vi "Config2Double.vi"(10 "Numeric in":u32, 11 "Config Address":T1 items=["ID", "Mode", "Baudrate", "Homing Offset", "Id P gain", "Id I gain", "Id D gain", "Iq P gain", "Iq I gain", "Iq D gain", "Velo P gain", "Velo I gain", "Velo D gain", "Posi P gain", "Posi I gain", "Posi D gain", "DirectForce P", "DirectForce I", "DirectForce D", "Limit Id Max", "Limit Iq Max", "Limit Velo Max", "Limit Posi Min", "Limit Posi Max", "Voltage Min", "Voltage Max", "Watchdog", "Temperature Low", "Temperature High"]) -> (3 "Numeric out":dbl)   [LabVIEW 2016, in "REV_2.lvlib"]
uses:
  REV_2.lvlib
  REV2_Config_Addr.ctl
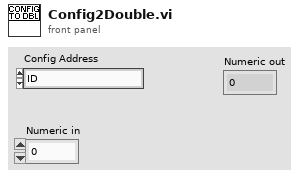
[diagram p1: front panel]
types:
  T1 = typedef "REV_2.lvlib/REV2_Config_Addr.ctl" = u8
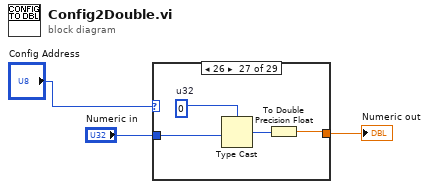
[diagram p0: block diagram]
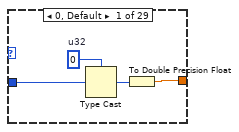
[diagram p2: hidden frame]
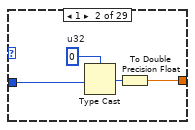
[diagram p3: hidden frame]
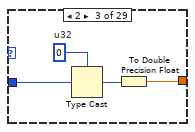
[diagram p4: hidden frame]
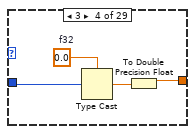
[diagram p5: hidden frame]
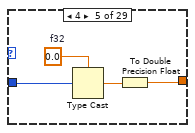
[diagram p6: hidden frame]
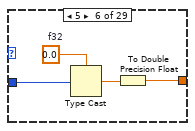
[diagram p7: hidden frame]
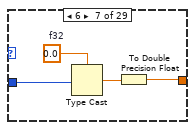
[diagram p8: hidden frame]
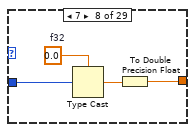
[diagram p9: hidden frame]
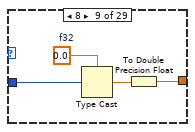
[diagram p10: hidden frame]
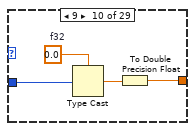
[diagram p11: hidden frame]
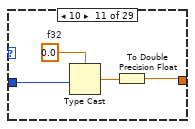
[diagram p12: hidden frame]
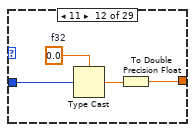
[diagram p13: hidden frame]
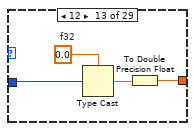
[diagram p14: hidden frame]
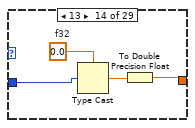
[diagram p15: hidden frame]
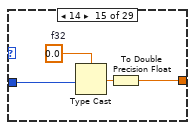
[diagram p16: hidden frame]
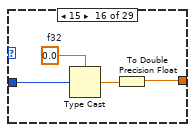
[diagram p17: hidden frame]
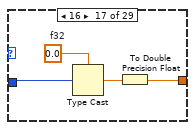
[diagram p18: hidden frame]
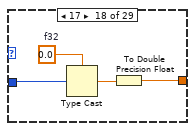
[diagram p19: hidden frame]
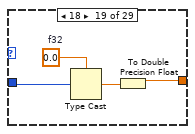
[diagram p20: hidden frame]
diagram:
  n1 = case shown="26" "Config Address" {
    tunnel: "Numeric in" -> [w6 w9 w14 w16 w21 w25 w29 w33 w37 w41 w45 w49 w52 w56 w61 w65 w68 w72 w76 w81 w85 w89 w93 w97 w101 w105 w110 w113 w117]
    tunnel: [w4 w8 w13 w17 w20 w24 w28 w32 w36 w40 w44 w48 w53 w57 w62 w64 w69 w73 w77 w80 w84 w88 w92 w96 w100 w104 w109 w112 w116] -> w3
    frame 0, Default {
      w7 = u32 0  # u32
      n2 = Type Cast(type=w7, x=w6) -> (*(type *) &x=w5:u32)
      n3 = To Double Precision Float(number=w5) -> (double precision float=w4:dbl)
    }
    frame 1 {
      w10 = u32 0  # u32
      n4 = Type Cast(type=w10, x=w9) -> (*(type *) &x=w11:u32)
      n5 = To Double Precision Float(number=w11) -> (double precision float=w8:dbl)
    }
    frame 2 {
      w12 = u32 0  # u32
      n6 = Type Cast(type=w12, x=w14) -> (*(type *) &x=w15:u32)
      n7 = To Double Precision Float(number=w15) -> (double precision float=w13:dbl)
    }
    frame 3 {
      w19 = sgl 0.0  # f32
      n8 = Type Cast(type=w19, x=w16) -> (*(type *) &x=w18:sgl)
      n9 = To Double Precision Float(number=w18) -> (double precision float=w17:dbl)
    }
    frame 4 {
      w23 = sgl 0.0  # f32
      n10 = Type Cast(type=w23, x=w21) -> (*(type *) &x=w22:sgl)
      n11 = To Double Precision Float(number=w22) -> (double precision float=w20:dbl)
    }
    frame 5 {
      w27 = sgl 0.0  # f32
      n12 = Type Cast(type=w27, x=w25) -> (*(type *) &x=w26:sgl)
      n13 = To Double Precision Float(number=w26) -> (double precision float=w24:dbl)
    }
    frame 6 {
      w31 = sgl 0.0  # f32
      n14 = Type Cast(type=w31, x=w29) -> (*(type *) &x=w30:sgl)
      n15 = To Double Precision Float(number=w30) -> (double precision float=w28:dbl)
    }
    frame 7 {
      w35 = sgl 0.0  # f32
      n16 = Type Cast(type=w35, x=w33) -> (*(type *) &x=w34:sgl)
      n17 = To Double Precision Float(number=w34) -> (double precision float=w32:dbl)
    }
    frame 8 {
      w39 = sgl 0.0  # f32
      n18 = Type Cast(type=w39, x=w37) -> (*(type *) &x=w38:sgl)
      n19 = To Double Precision Float(number=w38) -> (double precision float=w36:dbl)
    }
    frame 9 {
      w43 = sgl 0.0  # f32
      n20 = Type Cast(type=w43, x=w41) -> (*(type *) &x=w42:sgl)
      n21 = To Double Precision Float(number=w42) -> (double precision float=w40:dbl)
    }
    frame 10 {
      w46 = sgl 0.0  # f32
      n22 = Type Cast(type=w46, x=w45) -> (*(type *) &x=w47:sgl)
      n23 = To Double Precision Float(number=w47) -> (double precision float=w44:dbl)
    }
    frame 11 {
      w51 = sgl 0.0  # f32
      n24 = Type Cast(type=w51, x=w49) -> (*(type *) &x=w50:sgl)
      n25 = To Double Precision Float(number=w50) -> (double precision float=w48:dbl)
    }
    frame 12 {
      w55 = sgl 0.0  # f32
      n26 = Type Cast(type=w55, x=w52) -> (*(type *) &x=w54:sgl)
      n27 = To Double Precision Float(number=w54) -> (double precision float=w53:dbl)
    }
    frame 13 {
      w59 = sgl 0.0  # f32
      n28 = Type Cast(type=w59, x=w56) -> (*(type *) &x=w58:sgl)
      n29 = To Double Precision Float(number=w58) -> (double precision float=w57:dbl)
    }
    frame 14 {
      w60 = sgl 0.0  # f32
      n30 = Type Cast(type=w60, x=w61) -> (*(type *) &x=w63:sgl)
      n31 = To Double Precision Float(number=w63) -> (double precision float=w62:dbl)
    }
    frame 15 {
      w66 = sgl 0.0  # f32
      n32 = Type Cast(type=w66, x=w65) -> (*(type *) &x=w67:sgl)
      n33 = To Double Precision Float(number=w67) -> (double precision float=w64:dbl)
    }
    frame 16 {
      w70 = sgl 0.0  # f32
      n34 = Type Cast(type=w70, x=w68) -> (*(type *) &x=w71:sgl)
      n35 = To Double Precision Float(number=w71) -> (double precision float=w69:dbl)
    }
    frame 17 {
      w74 = sgl 0.0  # f32
      n36 = Type Cast(type=w74, x=w72) -> (*(type *) &x=w75:sgl)
      n37 = To Double Precision Float(number=w75) -> (double precision float=w73:dbl)
    }
    frame 18 {
      w79 = sgl 0.0  # f32
      n38 = Type Cast(type=w79, x=w76) -> (*(type *) &x=w78:sgl)
      n39 = To Double Precision Float(number=w78) -> (double precision float=w77:dbl)
    }
    frame 19 {
      w83 = sgl 0.0  # f32
      n40 = Type Cast(type=w83, x=w81) -> (*(type *) &x=w82:sgl)
      n41 = To Double Precision Float(number=w82) -> (double precision float=w80:dbl)
    }
    frame 20 {
      w87 = sgl 0.0  # f32
      n42 = Type Cast(type=w87, x=w85) -> (*(type *) &x=w86:sgl)
      n43 = To Double Precision Float(number=w86) -> (double precision float=w84:dbl)
    }
    frame 21 {
      w91 = sgl 0.0  # f32
      n44 = Type Cast(type=w91, x=w89) -> (*(type *) &x=w90:sgl)
      n45 = To Double Precision Float(number=w90) -> (double precision float=w88:dbl)
    }
    frame 22 {
      w95 = sgl 0.0  # f32
      n46 = Type Cast(type=w95, x=w93) -> (*(type *) &x=w94:sgl)
      n47 = To Double Precision Float(number=w94) -> (double precision float=w92:dbl)
    }
    frame 23 {
      w99 = sgl 0.0  # f32
      n48 = Type Cast(type=w99, x=w97) -> (*(type *) &x=w98:sgl)
      n49 = To Double Precision Float(number=w98) -> (double precision float=w96:dbl)
    }
    frame 24 {
      w103 = sgl 0.0  # f32
      n50 = Type Cast(type=w103, x=w101) -> (*(type *) &x=w102:sgl)
      n51 = To Double Precision Float(number=w102) -> (double precision float=w100:dbl)
    }
    frame 25 {
      w107 = sgl 0.0  # f32
      n52 = Type Cast(type=w107, x=w105) -> (*(type *) &x=w106:sgl)
      n53 = To Double Precision Float(number=w106) -> (double precision float=w104:dbl)
    }
    frame 26 {
      w108 = u32 0  # u32
      n54 = Type Cast(type=w108, x=w110) -> (*(type *) &x=w111:u32)
      n55 = To Double Precision Float(number=w111) -> (double precision float=w109:dbl)
    }
    frame 27 {
      w115 = sgl 0.0  # f32
      n56 = Type Cast(type=w115, x=w113) -> (*(type *) &x=w114:sgl)
      n57 = To Double Precision Float(number=w114) -> (double precision float=w112:dbl)
    }
    frame 28 {
      w119 = sgl 0.0  # f32
      n58 = Type Cast(type=w119, x=w117) -> (*(type *) &x=w118:sgl)
      n59 = To Double Precision Float(number=w118) -> (double precision float=w116:dbl)
    }
  }
  "Numeric out" <- w3
